vi "VeristandStart.vi"(2 "error in (no error)":errorcluster) -> (0 "error out":errorcluster)   [LabVIEW 2015, in "MiscHelperVIs.lvlib"]
uses:
  MiscHelperVIs.lvlib
  <vilib>/Utility/sysdir.llb/System Directory Type.ctl
  <vilib>/NI Veristand/Execution/Workspace/NI_VS Workspace ExecutionAPI.lvlib
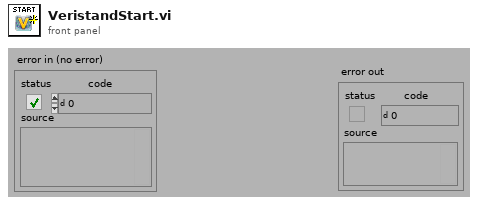
[diagram p1: front panel]
types:
  T1 = typedef "System Directory Type.ctl" = i32
  T2 = typedef "NI_VS Workspace ExecutionAPI.lvlib/WorkspaceAPI.ctl" = refnum<k24>
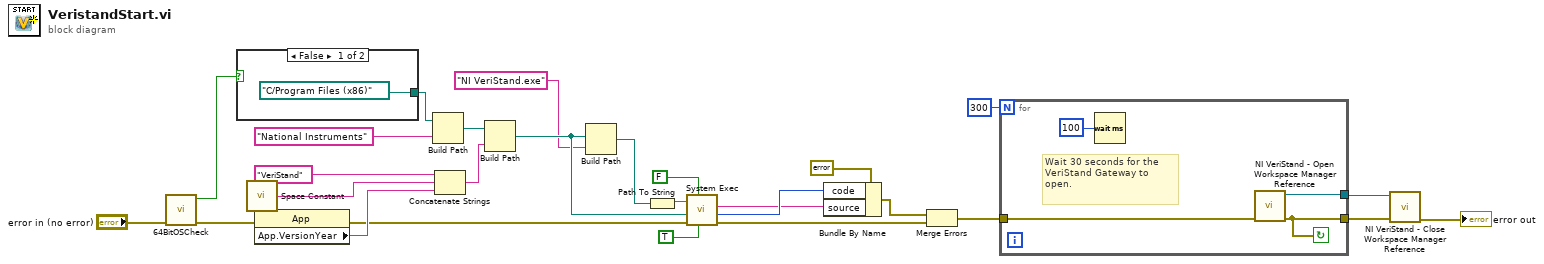
[diagram p0: block diagram]
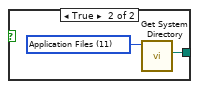
[diagram p2: hidden frame]
diagram:
  n1 = call "64BitOSCheck.vi"("error in (no error)"="error in (no error)") -> ("error out"=w6:errorcluster, "Is64Bit?"=w8:bool)  [unwired: 9 in]
  n2 = case shown="False" w8 {
    tunnel: [path "C:/Program Files (x86)" ("system directory") w29] -> w26
    frame False {
    }
    frame True {
      w30 = T1 11 items=["User Home"=0, "User Desktop"=1, "User Documents"=2, "User Application Data"=3, "User Preferences"=4, "User Temporary"=5, "Public Documents"=6, "Public Application Data"=7, "Public Preferences"=8, "Public Cache"=13, "System Core Libraries"=9, "System Installed Libraries"=10, "Application Files"=11, "Boot Volume Root"=12] ("system directory type")
      n3 = call <vilib>:"Get System Directory.vi"("system directory type"=w30) -> ("system directory"=w29:path)  [unwired: 10 in]
    }
  }
  n4 = call <vilib>:"Space Constant.vi"() -> ("String"=w19:string)
  n5 = property class="App"(error in=w6) -> (error out=w9:errorcluster, "App.VersionYear"=w20:string)  [unwired: 1 in, 1 out]
  n6 = Build Path(base path=w26, name or relative path="National Instruments") -> (appended path=w24:path)
  n7 = Concatenate Strings("VeriStand" ("name or relative path"), w19, w20) -> (w18:string)
  n8 = Build Path(base path=w24, name or relative path=w18) -> (appended path=w17:path)
  n9 = Build Path(base path=w17, name or relative path="NI VeriStand.exe") -> (appended path=w23:path)
  n10 = Path To String(path=w23) -> (string=w22:string)
  n11 = call <vilib>:"System Exec.vi"("run minimized? (F)"=TRUE, "wait until completion? (T)"=FALSE, "error in (no error)"=w9, "working directory"=w17, "command line"=w22) -> ("error out"=w12:errorcluster, "return code"=w14:i32, "standard error"=w11:string)  [unwired: 3 in, 1 out]
  n12 = Bundle By Name(cluster=errorcluster {"status"=FALSE, "code"=0, "source"=""} ("error in (no error)"), "code"=w14, "source"=w11) -> (w13:errorcluster)
  n13 = Merge Errors(w13, w12) -> (w3:errorcluster)
  n14 = for {
    N: 300 -> [_]
    tunnel: [w32] -> w1
    tunnel: w3 -> [w31]
    tunnel: [w33] -> w5
    stop <- w33 continue-if-true
    # "Wait 30 seconds for the VeriStand Gateway to open."
    n15 = Wait (ms)(milliseconds to wait=u32 100) -> ()  [unwired: 1 out]
    n16 = call <vilib>:"NI VeriStand - Open Workspace Manager Reference.vi"("error in (no error)"=w31) -> ("error out"=w33:errorcluster, "WorkspaceManager"=w32:T2)  [unwired: 9 in]
  }
  n17 = call <vilib>:"NI VeriStand - Close Workspace Manager Reference.vi"("error in (no error)"=w5, "WorkspaceManager"=w1) -> ("error out"=→"error out":errorcluster)  [unwired: 9 in]
